vi "APS absolute arc move.vi"(6 "Angle":i32, 7 "Max_Arc_Speed":i32, 8 "error in (no error)":errorcluster caption="错误输入（无错误）", 9 "Center_Pos_Array":i32, 10 "Axis_ID_Array":i32, 11 "Dimension":i32) -> (0 "error out":errorcluster caption="错误输出", 1 "Center_Pos_Array out":i32, 2 "Axis_ID_Array out":i32, 3 "function return":i32)   [LabVIEW 2011, in "APS168.lvlib"]
doc: "I32 FNTYPE APS_absolute_arc_move( I32 Dimension, I32 *Axis_ID_Array, I32 *Center_Pos_Array, I32 Max_Arc_Speed, I32 Angle );"
uses:
  APS168.lvlib
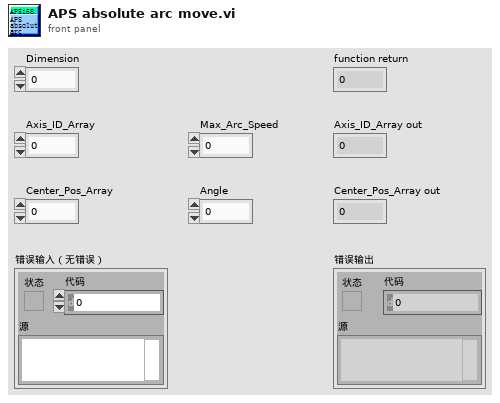
[diagram p1: front panel]
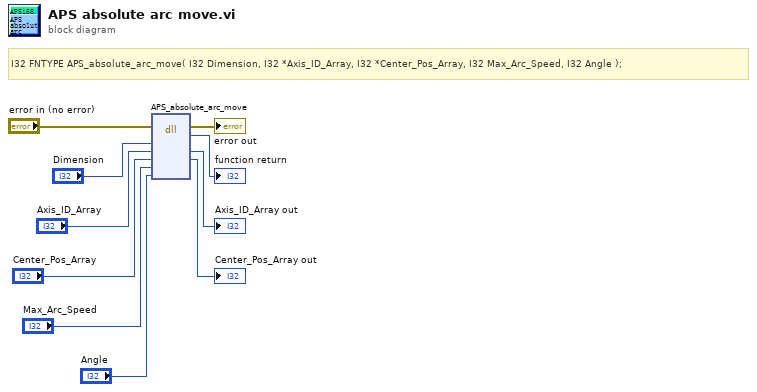
[diagram p0: block diagram]
diagram:
  # "I32 FNTYPE APS_absolute_arc_move( I32 Dimension, I32 *Axis_ID_Array, I32 *Center_Pos_Array, I32 Max_Arc_Speed, I32 Angle );"
  n1 = dll-call lib="PTH1Labs E软件ADLINK 204CAPS_1_7_1_LIB line 连续运动204APS168.*" fn="APS_absolute_arc_move"(error in="error in (no error)", "Dimension"="Dimension", "Axis_ID_Array"="Axis_ID_Array", "Center_Pos_Array"="Center_Pos_Array", "Max_Arc_Speed"="Max_Arc_Speed", "Angle"="Angle") -> (error out=→"error out":errorcluster, →"function return":i32, "Axis_ID_Array"=→"Axis_ID_Array out":i32, "Center_Pos_Array"=→"Center_Pos_Array out":i32)  [unwired: 5 in, 1 out]
